vi "Autosize All Table Columns (Uniform Text).vi"(6 "IngoreCols(Empty as default)":i32[](array[numeric]), 8 "error in (no error)":errorcluster, 10 "Array":string[][](array[string]), 11 "Control in":refnum<vi>) -> (0 "error out":errorcluster, 3 "Control in":refnum<vi>)   [LabVIEW 2017]
doc: "This VI resizes each column of the table specified by Table Ref based on the widest entry of the column. Additionally, if Resize Table? is TRUE, the VI will set the table width based on the number of populated columns."
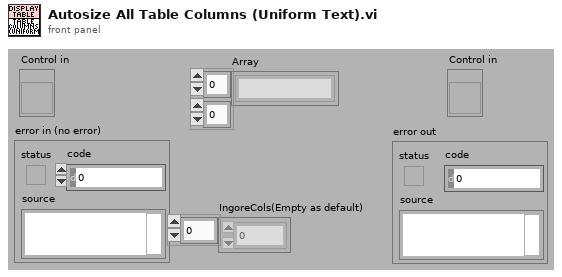
[diagram p1: front panel]
types:
  T1 = cluster{"Font Name:":string, "Size":i16, "Strikeout?":bool, "Italic?":bool, "Underline?":bool, "Outline?":bool, "Shadow?":bool, "Bold?":bool}
  T2 = enum16{"User-specified Font", "Application Font", "System Font", "Dialog Font"}
  T3 = cluster{"left":i16, "top":i16, "right":i16, "bottom":i16}
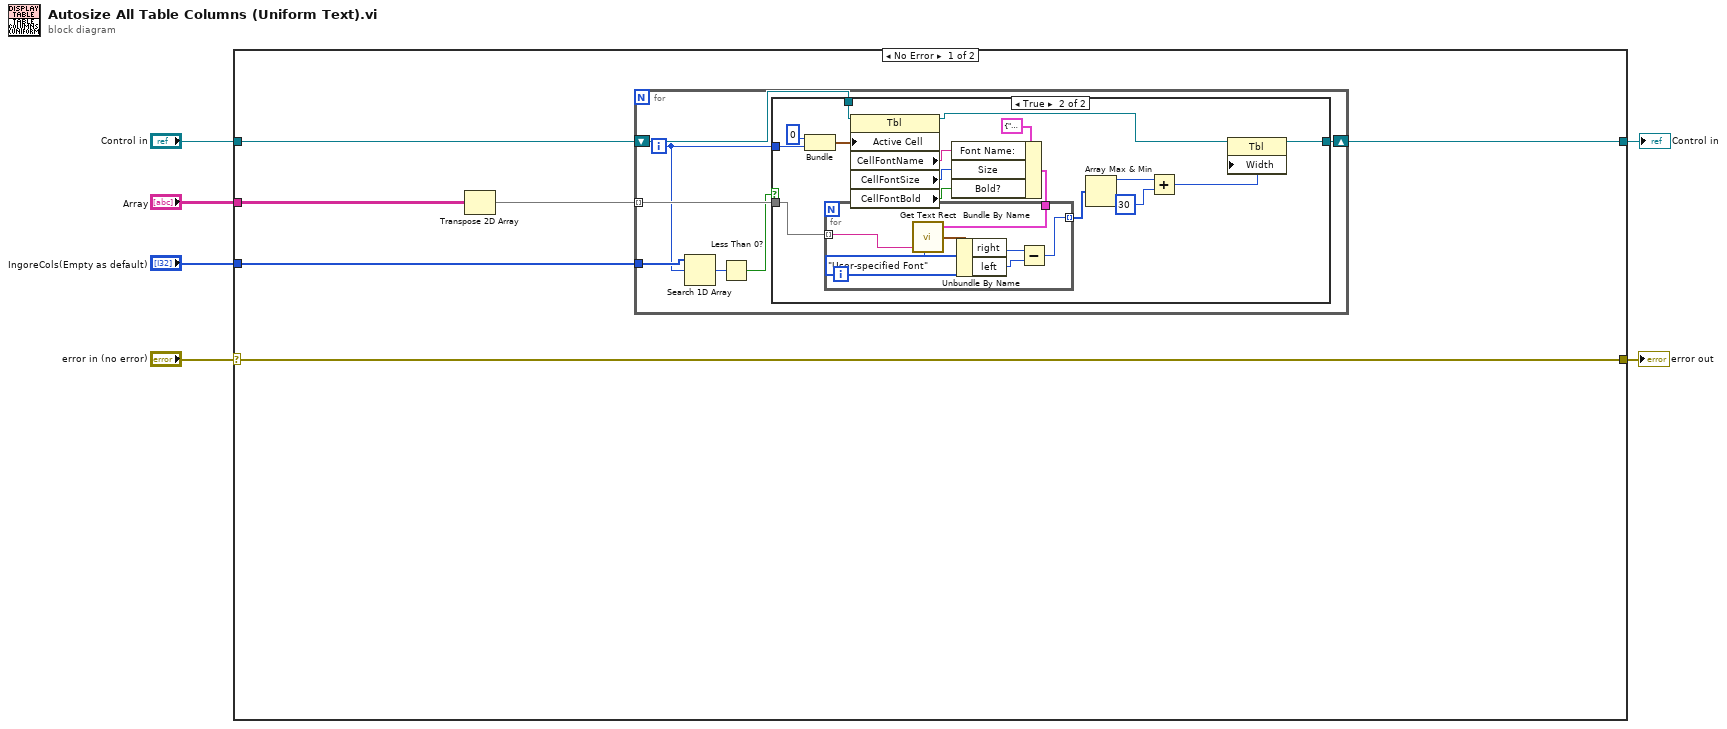
[diagram p0: block diagram]
diagram:
  n1 = case shown="No Error" "error in (no error)" {
    selector: "error in (no error)" -> [w9 w45]
    tunnel: "Control in" -> [w11 w44]
    tunnel: [w10 w44] -> w4
    tunnel: [w9 w45] -> w3
    tunnel: "Array" -> [w8 _]
    tunnel: "IngoreCols(Empty as default)" -> [w7 _]
    frame No Error {
      n2 = Transpose 2D Array(2D array=w8) -> (transposed array=w12:string[][])
      n3 = for {
        tunnel: w12 -> [w19] mode=indexing
        shift-right: [w17] -> w10
        shift-left: w11 -> [w18]
        tunnel: w7 -> [w16]
        i -> [w15]
        n4 = Search 1D Array(1D array=w16, element=w15) -> (index of element=w14:i32)  [unwired: 1 in]
        n5 = Less Than 0?(x=w14) -> (x < 0?=w13:bool)
        n6 = case shown="True" w13 {
          tunnel: w19 -> [_ w36]
          tunnel: w15 -> [_ w26]
          tunnel: w18 -> [w20 w27]
          tunnel: [w20 w23] -> w17
          frame False {
          }
          frame True {
            n7 = Bundle(0, w26) -> (w22:cluster{i32, i32})  [unwired: 1 in]
            n8 = property class="Tbl"(reference=w27, "Active Cell"=w22) -> (reference out=w24:refnum<vi>, "CellFontName"=w31:string, "CellFontSize"=w29:u32, "CellFontBold"=w30:bool)  [unwired: 1 in, 1 out]
            n9 = Bundle By Name(cluster=T1 {"Font Name:"="", "Size"=0, "Strikeout?"=FALSE, "Italic?"=FALSE, "Underline?"=FALSE, "Outline?"=FALSE, "Shadow?"=FALSE, "Bold?"=FALSE} ("[user-specified font]"), "Font Name:"=w31, "Size"=w29, "Bold?"=w30) -> (w25:T1)
            n10 = for {
              tunnel: w36 -> [w43] mode=indexing
              tunnel: [w39] -> w35 mode=indexing
              tunnel: w25 -> [w38]
              n11 = call <vilib>:"Get Text Rect.vi"("desired font(Application)"=T2."User-specified Font", "text"=w43, "[user-specified font]"=w38) -> ("rect"=w42:T3)  [unwired: 6 in]
              n12 = Unbundle By Name(w42) -> ("right"=w41:i16, "left"=w40:i16)
              n13 = Subtract(x=w41, y=w40) -> (x-y=w39:i16)
            }
            n14 = Array Max & Min(array=w35) -> (max value=w32:i16)  [unwired: 3 out]
            n15 = Add(x=w32, y=i16 30) -> (x+y=w33:i16)
            n16 = property on="Property Node" class="Tbl"(reference=w24, "Width"=w33) -> (reference out=w23:refnum<vi>)  [unwired: 1 in, 1 out]
          }
        }
      }
    }
    frame Error {
    }
  }
  "error out" <- w3
  "Control in" <- w4
